vi "DPT Panel Dryer PreCondition.vi"(0 "Test Fixture Hardware":T1={"Power "={"Yokogawa"={"WT210"={"Sample Rate (1: 0.25s)"=1, "A Range (12: 20A)"=11, "V Range (6: 600V)"=4, "Power VISA Yokogawa WT210"="WT210"}, "WT500"={"Power VISA Yokogawa WT500"="", "V Range (8: 1000V)"=6, "I Range (7: 40A)"=7, "Update Rate (3: 500ms)"=2}, "WT310_2"={"Sample Rate (1: 0.25s)"=1, "A Range (12: 20A)"=11, "V Range (6: 600V)"=4, "Power VISA Yokogawa WT310_2"="WT310_2"}, "WT310_3"={"Sample Rate (1: 0.25s)"=1, "A Range (12: 20A)"=11, "V Range (6: 600V)"=4, "Power VISA Yokogawa WT310_3"="WT310_3"}}, "Aplus"={"Aplus IP Address"="192.168.1.101", "Remote Port"=502, "Instrument"="APLUS", "Instr Driver Revision"="1.03.0053"}, "Power Limits"={"Crest Factor"={"Upper Limit"=1.49, "Lower Limit"=1.34}, "Harmonic Content"={"Uthd"=2.0}, "Voltage"={"% Error"=2.0}, "Stability"={"<1 Watt "={"Wattage"=1.0, "Slope (mW/H)"=10.0}, ">1 Watt"={"1%Power/Hour"=1.0}}}, "Nominal Voltage"=120, "Time Limit (s)"=10800.0, "Power Variation Limit (%)"=50.0, "Power Supply"={"Chroma 61605"="CHROMA", "Use Chroma?"=FALSE}}, "Weight Scale"={"Com Options"={"IND560Scale VISA"="IND560", "IP Address"="", "Remote Port"=502, "Setra Scale VISA"="SETRA", "GSE 350"="GSE350"}, "Select Scale"=""}, "Flow Rates"={"Laurel Cold IP Address"="", "Laurel Hot IP Address"="", "Hot Water Laurel VISA"="LaurelMeter_Hot", "Cold Water Laurel VISA"="LaurelMeter_Cold", "Remote Port"=0, "Laurel Communication Type"="", "Meters To Collect (Hot Cold)"="", "HOT Laurel Reference"=refnum, "COLD Laurel Reference"=refnum}, "Analog Data"={"Agilent"={"Agilent 34972_1"="34972A_1", "Agilent 34972_2"="34972A_2", "Agilent 34972_3"="34972A_3", "Agilent 34972_4"="34972A_3", "Agilent 34972_5"="34972A_3", "Agilent 34972_6"="34972A_3", "Agilent Gain"=0.0, "TC Type (K,J,T)"="", "Instrument IDN?"="", "TC Channels-List"="", "Analog Channels-List"="", "Agilent Cluster Array"=[], "TC Channels-List 2"="", "Analog Channels-List 2"=""}, "Yokogawa"={"MW100"="MW100", "Intellifaucet"=FALSE}, "Select Analog"="", "TC Coefficients"={"TC Coefficients 1"=[], "TC Coefficients 2"=[], "TC Coefficients 3"=[], "TC Coefficients 4"=[], "TC Coefficients 5"=[], "TC Coefficients 6"=[], "TC Coefficients 7"=[]}, "NI Tasks (Dryer DOE)"=["TC Temps-Module 1", "TC Temps-Module 2", "TC Temps-Module 3", "TC Temps-Module 4", "TC Temps-Module 5", "Gas and Temp-Module 6", "AC_DC Events-Module 7"], "Laurel Analog"={"Laurel IP (Water Temp)"="", "Laurel IP (Pressure)"=""}}, "ITHX-Temp Humidity"={"IP Address 1"="", "Remote Port"=0, "IP Address 2"="", "IP Address 3"=""}, "Gas Meter COM Ports"={"Gas Meter 1"="COM3", "Gas Meter 2"="COM4", "Gas Meter 3"="COM5", "Gas Meter 4"="COM6", "Gas Meter 5"="COM7", "Gas Meter 6"="COM8"}, "Barometric Pressure"={"HEISE 901A"="HEISE", "Use Barometer?"=FALSE}} {"Power"."Yokogawa"."WT310_3"."V Range (6: 600V)" items=["Auto", "15V", "30V", "60V", "150V", "300V", "600V"]; "Power"."Yokogawa"."WT310_3"."A Range (12: 20A)" items=["Auto", "5mA", "10mA", "20mA", "50mA", "100mA", "200mA", "0.5A", "1A", "2A", "5A", "10A", "20A", "50mV", "100mV", "200mV", "2.5V", "5V", "10V"]; "Power"."Yokogawa"."WT310_3"."Sample Rate (1: 0.25s)" items=["0.1s", "0.25s", "0.5s", "1s", "2s", "5s"]; "Power"."Yokogawa"."WT310_2"."V Range (6: 600V)" items=["Auto", "15V", "30V", "60V", "150V", "300V", "600V"]; "Power"."Yokogawa"."WT310_2"."A Range (12: 20A)" items=["Auto", "5mA", "10mA", "20mA", "50mA", "100mA", "200mA", "0.5A", "1A", "2A", "5A", "10A", "20A", "50mV", "100mV", "200mV", "2.5V", "5V", "10V"]; "Power"."Yokogawa"."WT310_2"."Sample Rate (1: 0.25s)" items=["0.1s", "0.25s", "0.5s", "1s", "2s", "5s"]; "Power"."Yokogawa"."WT500"."Update Rate (3: 500ms)" items=["-", "100ms", "200ms", "500ms", "1s", "2s", "5s"]; "Power"."Yokogawa"."WT500"."I Range (7: 40A)" items=["AUTO", "500 mA", "1 A", "2 A", "5 A", "10 A", "20 A", "40 A", "S-AUTO", "50 mV", "100 mV", "200 mV", "500 mV", "1 V", "2 V", "5 V", "10 V", "250 mA", "500 mA", "1 A", "2.5 A", "5 A", "10 A", "20 A", "25 mV", "50 mV", "100 mV", "250 mV", "500 mV", "1 V", "2.5 V", "5 V"]; "Power"."Yokogawa"."WT500"."V Range (8: 1000V)" items=["AUTO", "15", "30", "60", "100", "150", "300", "600", "1000", "7.5", "15", "30", "50", "75", "150", "300", "500"]; "Power"."Yokogawa"."WT210"."V Range (6: 600V)" items=["Auto", "15V", "30V", "60V", "150V", "300V", "600V"]; "Power"."Yokogawa"."WT210"."A Range (12: 20A)" items=["Auto", "5mA", "10mA", "20mA", "50mA", "100mA", "200mA", "0.5A", "1A", "2A", "5A", "10A", "20A", "50mV", "100mV", "200mV", "2.5V", "5V", "10V"]; "Power"."Yokogawa"."WT210"."Sample Rate (1: 0.25s)" items=["0.1s", "0.25s", "0.5s", "1s", "2s", "5s"]}, 7 "Power On Threshold":dbl=25.0, 11 "Error In":errorcluster) -> (4 "Cold Dryer Weight":dbl, 15 "Error Out":errorcluster)   [LabVIEW 2018]
uses:
  Utility/Custom Pallet Controls/Custom Pallet String.ctl
  Utility/Custom Pallet Controls/Custom Pallet DBL.ctl
  Utility/Custom Pallet Controls/Custom Pallet Timer.ctl
  Washer DOE/Type Definitions/DOE Test Fixture Hardware.ctl
  Utility/Type Definitions/UTILITY Power Inputs Control.ctl
  Drivers/IND560 Scale Monitor/Type Definitions/IND560 Configuration.ctl
  Hybrid Water Heater/Type Definitions/HEWH Agilent Cluster.ctl
  Utility/Type Definitions/UTILITY TC Coefficients.ctl
  Drivers/Omega FMA-1600A Series Gas Flow Meter/Type Definitions/FMA1600A COM Ports.ctl
  Washer DOE/Type Definitions/DOE Dryer NI Card Settings.ctl
panel:
  out "RDB F":dbl(graph)
  in  "Tab Control":enum32{"Page 1", "Page 2"}(tab)
  out "15 min Up":bool
  out "Temp stable":bool
  out "Current State":string
  in  "Debug?":bool=TRUE
  in  "10 Min":i32=600
  in  "5min":dbl=300.0
  out "T0":dbl
  out "Tstart 5min":dbl
  out "Tstart 10min":dbl
  out "Debug State":string[](array[string])
  out "Power Greater Than Threshold":bool
  out "Timer":T7 format="%<%H:%M:%S>t"
  out "TC 1 - RDB (°F)":T8 format="%.2f"
  out "Ambient Temp(F)":T8 format="%.2f"
  out "Relative Humidity":T8 format="%.2f"
  out "Power (Watts)":T8 format="%.2f"
  out "Board ID":T9
  in  "Exit":bool
  # "Before any test cycle, operate the dryer without a test load in the non-heat mode for 15 minutes\nor until the discharge air temperature is varying less than 1 °F for 10 minutes, which ever is longer, in the test installation location\nwith the ambient conditions within the specified rest condition tolerances of 2.2."
  # "2.2 Ambient temperature and humidity. Maintain the room ambient air temperature at 75 ±3 °F and the room relative humidity at 50\n±10 percent relative humidity"
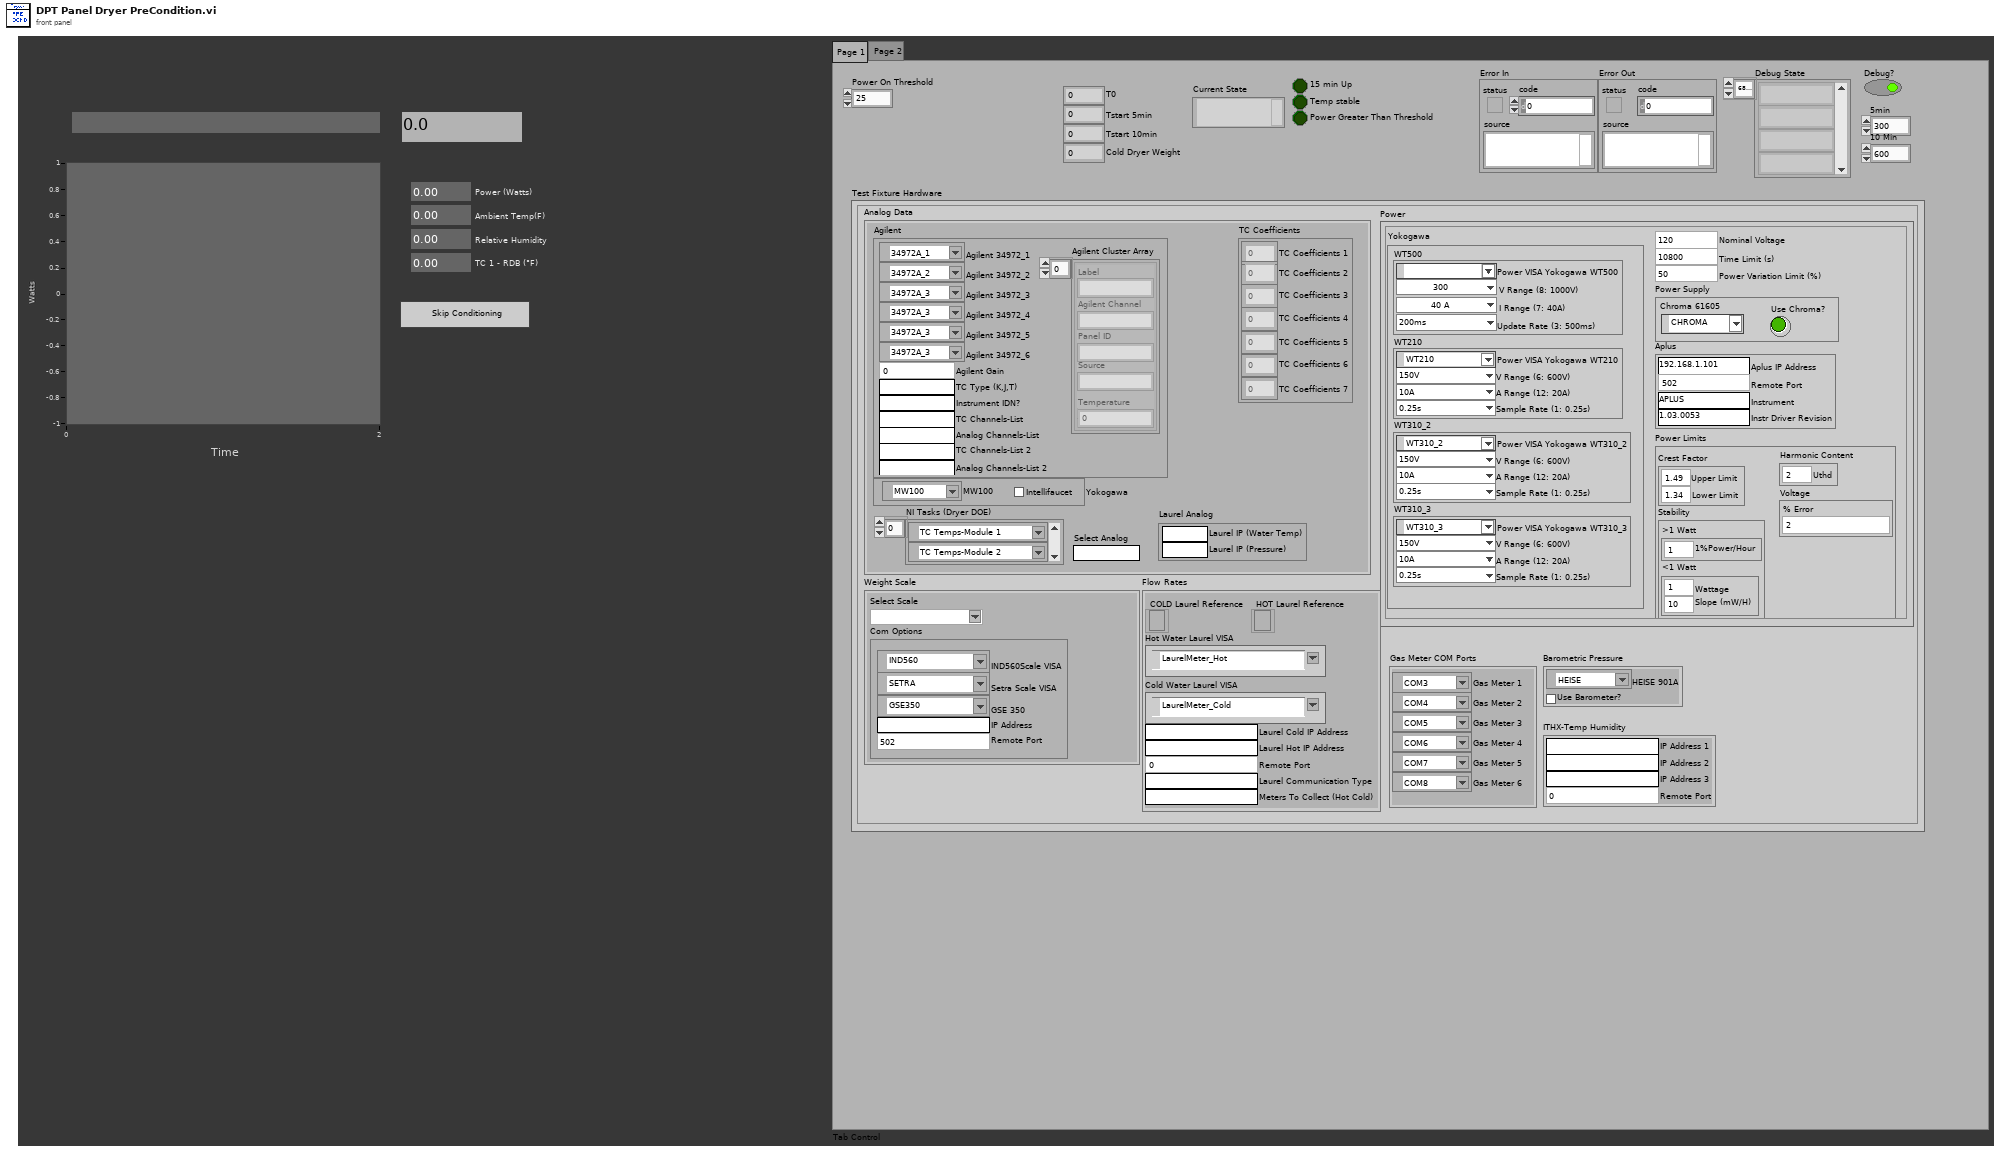
[diagram p1: front panel]
types:
  T1 = typedef "DOE Test Fixture Hardware.ctl" = cluster{"Power ":T2, "Weight Scale":cluster{"Com Options":T3, "Select Scale":string}, "Flow Rates":cluster{"Laurel Cold IP Address":string, "Laurel Hot IP Address":string, "Hot Water Laurel VISA":refnum<visa-resource-name>, "Cold Water Laurel VISA":refnum<visa-resource-name>, "Remote Port":u16, "Laurel Communication Type":string, "Meters To Collect (Hot Cold)":string, "HOT Laurel Reference":refnum<k5>, "COLD Laurel Reference":refnum<k5>}, "Analog Data":cluster{"Agilent":cluster{"Agilent 34972_1":refnum<visa-resource-name>, "Agilent 34972_2":refnum<visa-resource-name>, "Agilent 34972_3":refnum<visa-resource-name>, "Agilent 34972_4":refnum<visa-resource-name>, "Agilent 34972_5":refnum<visa-resource-name>, "Agilent 34972_6":refnum<visa-resource-name>, "Agilent Gain":dbl, "TC Type (K,J,T)":string, "Instrument IDN?":string, "TC Channels-List":string, "Analog Channels-List":string, "Agilent Cluster Array":T4[], "TC Channels-List 2":string, "Analog Channels-List 2":string}, "Yokogawa":cluster{"MW100":refnum<visa-resource-name>, "Intellifaucet":bool}, "Select Analog":string, "TC Coefficients":T5, "NI Tasks (Dryer DOE)":refnum<k21>[], "Laurel Analog":cluster{"Laurel IP (Water Temp)":string, "Laurel IP (Pressure)":string}}, "ITHX-Temp Humidity":cluster{"IP Address 1":string, "Remote Port":u16, "IP Address 2":string, "IP Address 3":string}, "Gas Meter COM Ports":T6, "Barometric Pressure":cluster{"HEISE 901A":refnum<visa-resource-name>, "Use Barometer?":bool}}
  T2 = typedef "UTILITY Power Inputs Control.ctl" = cluster{"Yokogawa":cluster{"WT210":cluster{"Sample Rate (1: 0.25s)":i32, "A Range (12: 20A)":i32, "V Range (6: 600V)":i32, "Power VISA Yokogawa WT210":refnum<visa-resource-name>}, "WT500":cluster{"Power VISA Yokogawa WT500":refnum<visa-resource-name>, "V Range (8: 1000V)":i32, "I Range (7: 40A)":i32, "Update Rate (3: 500ms)":i32}, "WT310_2":cluster{"Sample Rate (1: 0.25s)":i32, "A Range (12: 20A)":i32, "V Range (6: 600V)":i32, "Power VISA Yokogawa WT310_2":refnum<visa-resource-name>}, "WT310_3":cluster{"Sample Rate (1: 0.25s)":i32, "A Range (12: 20A)":i32, "V Range (6: 600V)":i32, "Power VISA Yokogawa WT310_3":refnum<visa-resource-name>}}, "Aplus":cluster{"Aplus IP Address":string, "Remote Port":i32, "Instrument":string, "Instr Driver Revision":string}, "Power Limits":cluster{"Crest Factor":cluster{"Upper Limit":dbl, "Lower Limit":dbl}, "Harmonic Content":cluster{"Uthd":dbl}, "Voltage":cluster{"% Error":dbl}, "Stability":cluster{"<1 Watt ":cluster{"Wattage":dbl, "Slope (mW/H)":dbl}, ">1 Watt":cluster{"1%Power/Hour":dbl}}}, "Nominal Voltage":i32, "Time Limit (s)":dbl, "Power Variation Limit (%)":dbl, "Power Supply":cluster{"Chroma 61605":refnum<visa-resource-name>, "Use Chroma?":bool}}
  T3 = typedef "IND560 Configuration.ctl" = cluster{"IND560Scale VISA":refnum<visa-resource-name>, "IP Address":string, "Remote Port":u16, "Setra Scale VISA":refnum<visa-resource-name>, "GSE 350":refnum<visa-resource-name>}
  T4 = typedef "HEWH Agilent Cluster.ctl" = cluster{"Label":string, "Agilent Channel":string, "Panel ID":string, "Source":string, "Temperature":dbl}
  T5 = typedef "UTILITY TC Coefficients.ctl" = cluster{"TC Coefficients 1":dbl[], "TC Coefficients 2":dbl[], "TC Coefficients 3":dbl[], "TC Coefficients 4":dbl[], "TC Coefficients 5":dbl[], "TC Coefficients 6":dbl[], "TC Coefficients 7":dbl[]}
  T6 = typedef "FMA1600A COM Ports.ctl" = cluster{"Gas Meter 1":refnum<visa-resource-name>, "Gas Meter 2":refnum<visa-resource-name>, "Gas Meter 3":refnum<visa-resource-name>, "Gas Meter 4":refnum<visa-resource-name>, "Gas Meter 5":refnum<visa-resource-name>, "Gas Meter 6":refnum<visa-resource-name>}
  T7 = typedef "Custom Pallet Timer.ctl" = dbl
  T8 = typedef "Custom Pallet DBL.ctl" = dbl
  T9 = typedef "Custom Pallet String.ctl" = string
  T10 = enum32{"invalid app kind", "Development System", "Run Time System", "Student Edition", "Embedded LabVIEW", "Evaluation", "Custom"}
  T11 = enum32{"Invalid", "Standard", "Closed", "Hidden", "Minimized", "Maximized"}
  T12 = typedef "DOE Dryer NI Card Settings.ctl" = cluster{"Disable NI Card 1":bool, "Disable NI Card 2":bool, "Disable NI Card 3":bool, "Disable NI Card 4":bool, "Disable NI Card 5":bool, "Disable NI Card 6":bool, "Disable NI Card 7":bool}
  T13 = cluster{"Core":cluster{"Current VI Reference":refnum<vi>, "Close Panel on Exit?":bool}, "Agilent Channel List":string, "Power On Threshold":dbl, "T0":dbl, "Tstart":dbl, "Temps":dbl[], "Test Fixture Hardware":T1}
  T14 = cluster{"Current VI Reference":refnum<vi>, "Close Panel on Exit?":bool}
  T15 = typedef "UTILITY Power Data.ctl" = cluster{"Current (A):Element 1":dbl, "Current (A):Element 2":dbl, "Power (W):Sigma":dbl, "Watt Hours (Wh):Sigma":dbl, "Voltage (V):Element 2":dbl, "Voltage (V):Element 1":dbl, "Current Crest Factor:Element 1":dbl, "Current Crest Factor:Element 2":dbl, "Voltage Harmonic (%):Element 1":dbl, "Voltage Harmonic (%):Element 2":dbl, "Voltage Crest Factor:Element 1":dbl, "Voltage Crest Factor:Element 2":dbl, "Time:Element 1":dbl, "Frequency (Hz):Element 1":dbl, "Apparent Power (VA):Element 1":dbl, "Apparent Power (VA):Element 2":dbl, "Power Factor:Element 1":dbl, "Power Factor:Element 2":dbl, "Max Watt Hours":dbl, "Voltage (V):Element 2 Avg":dbl, "Voltage (V):Element 1 Avg":dbl}
  T16 = typedef "iBTHX Data Values.ctl" = cluster{"iBTHX Barometric Pressure (mbar/hPa)":dbl, "iBTHX Humidity (%)":dbl, "iBTHX Temperature (°F)":dbl, "iBTHX DewPoint Temp":dbl}
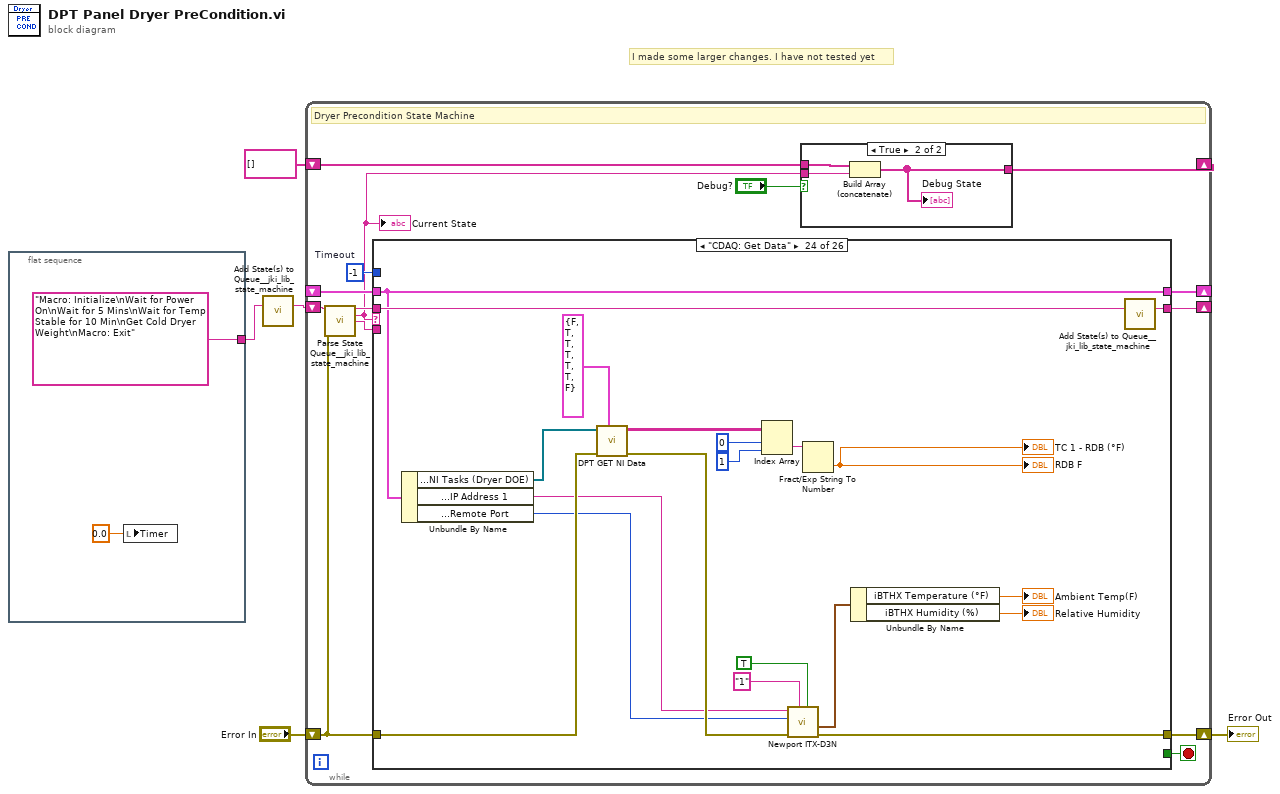
[diagram p0: block diagram]
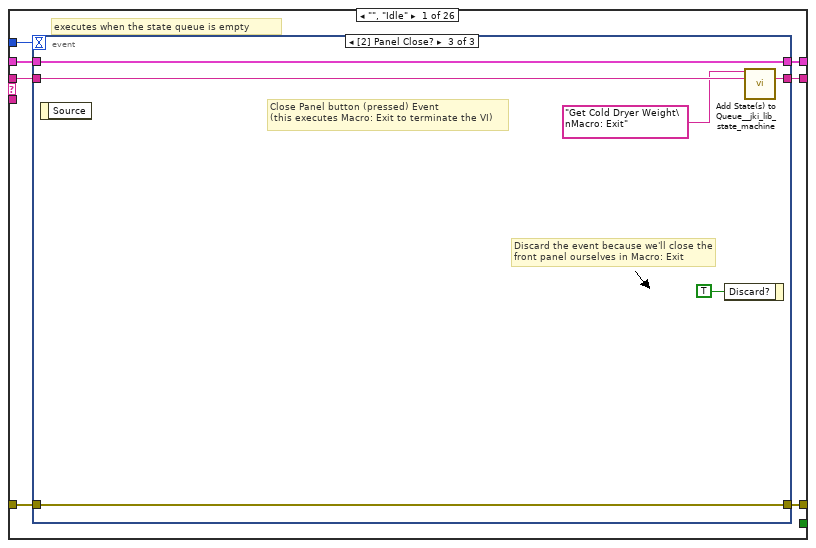
[diagram p3: hidden frame]
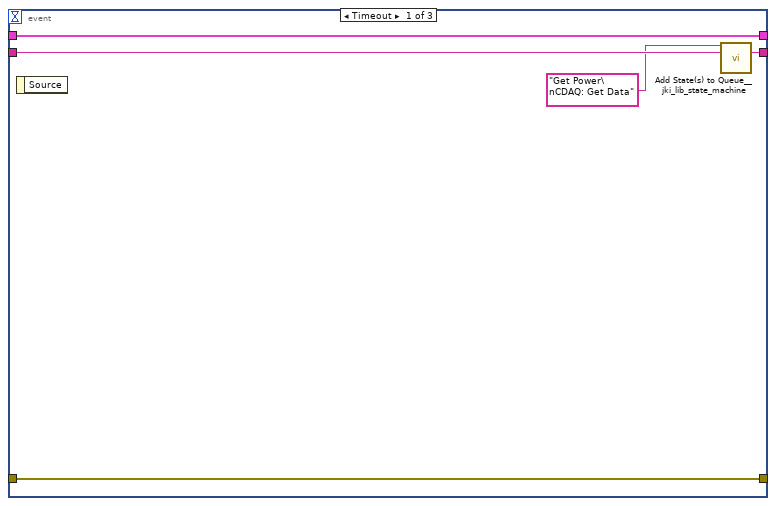
[diagram p4: hidden frame]
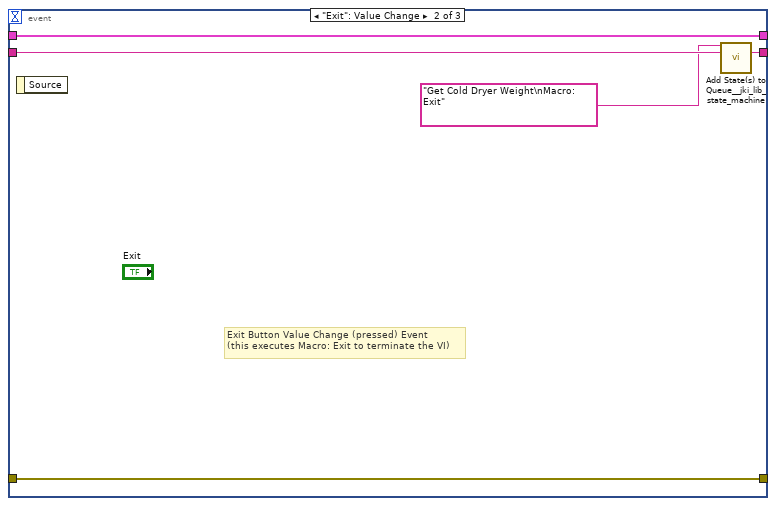
[diagram p5: hidden frame]
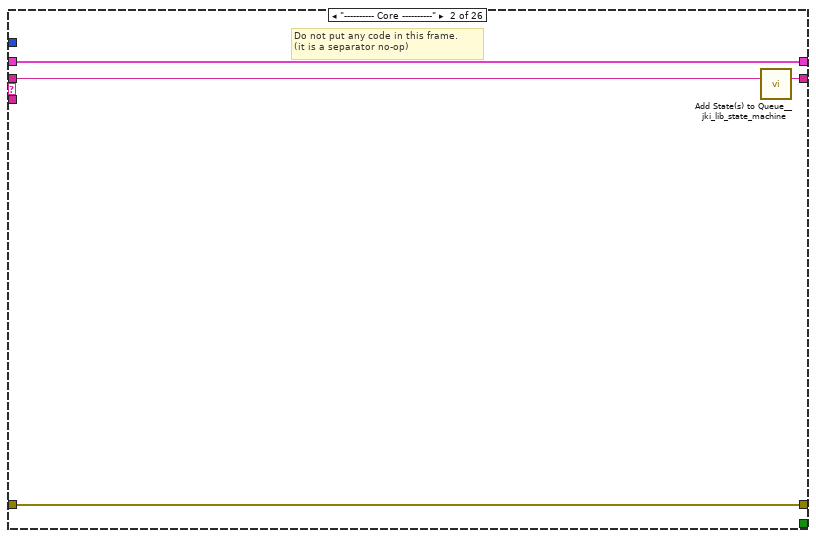
[diagram p6: hidden frame]
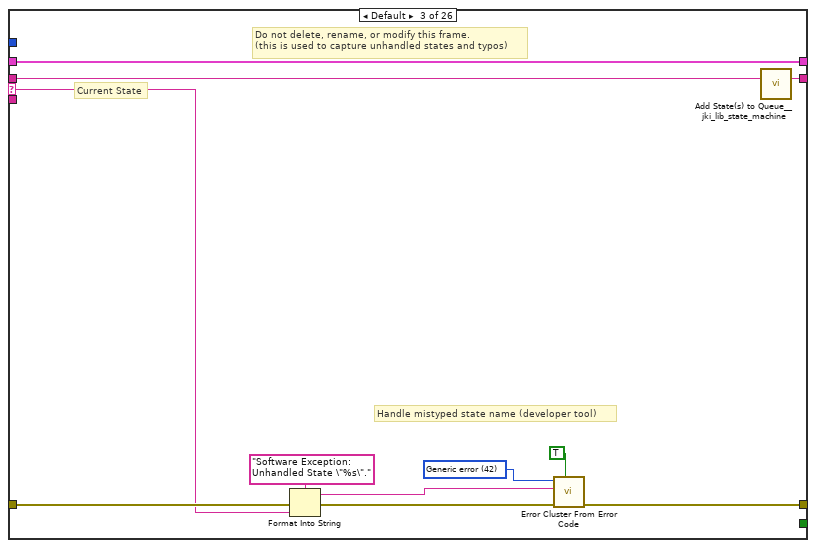
[diagram p7: hidden frame]
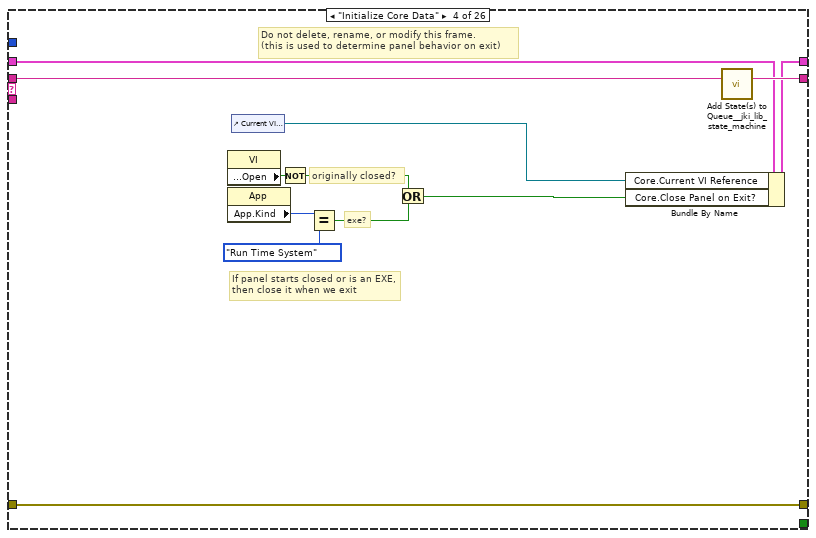
[diagram p8: hidden frame]
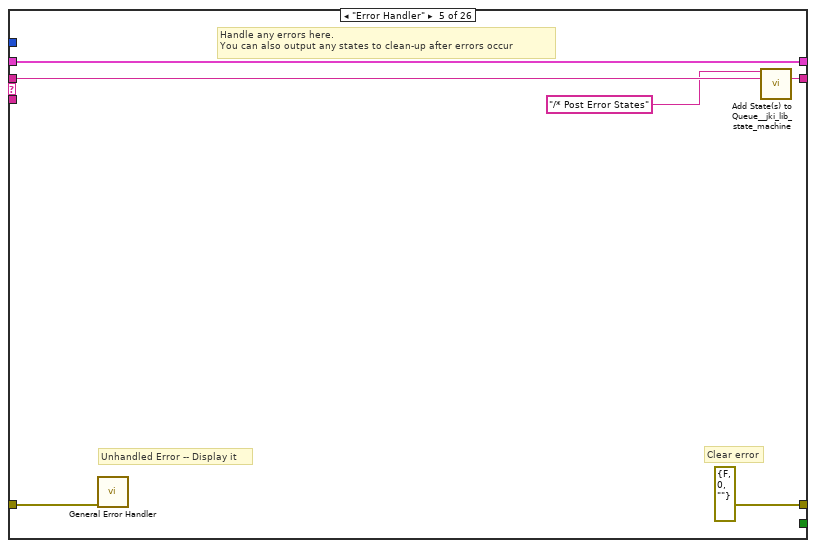
[diagram p9: hidden frame]
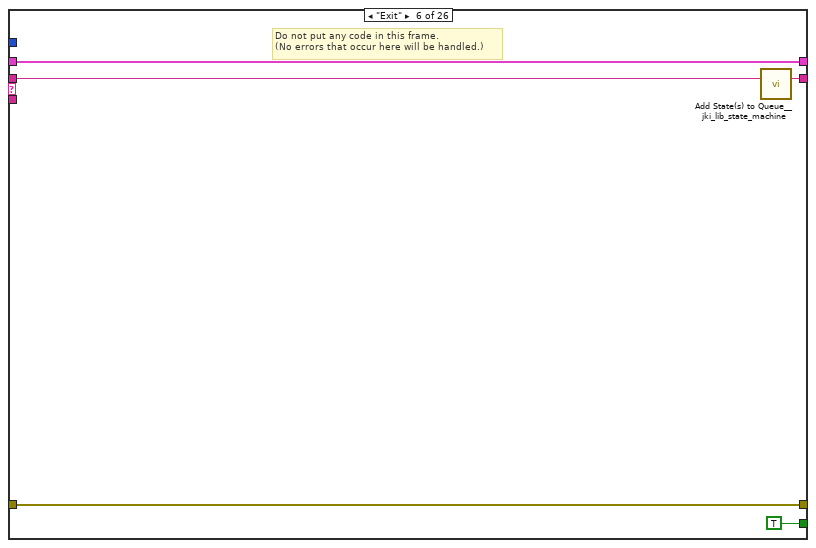
[diagram p10: hidden frame]
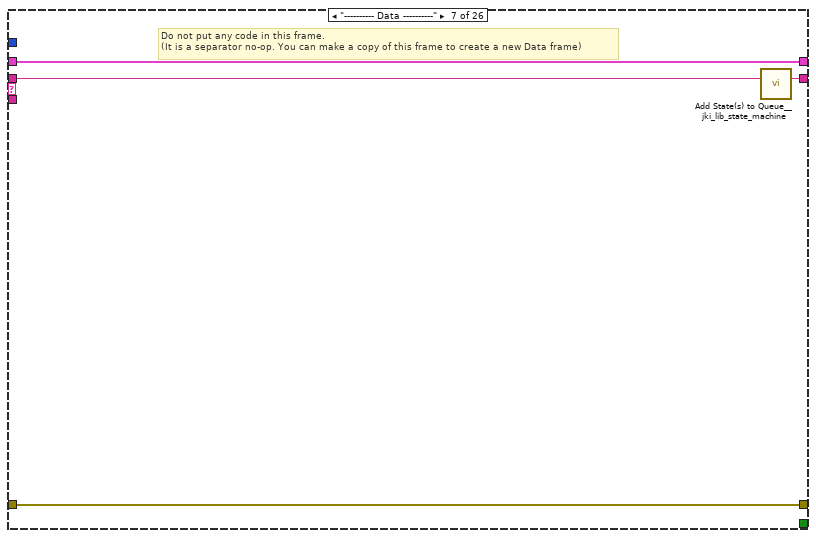
[diagram p11: hidden frame]
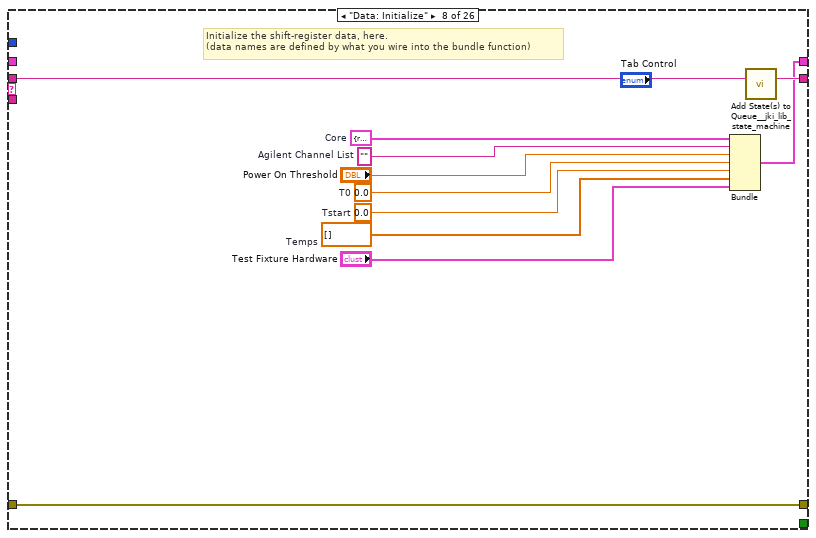
[diagram p12: hidden frame]
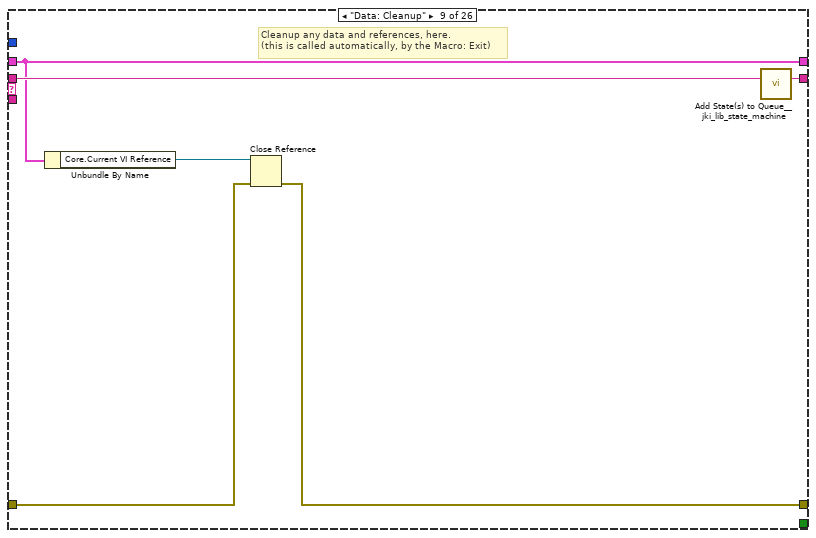
[diagram p13: hidden frame]
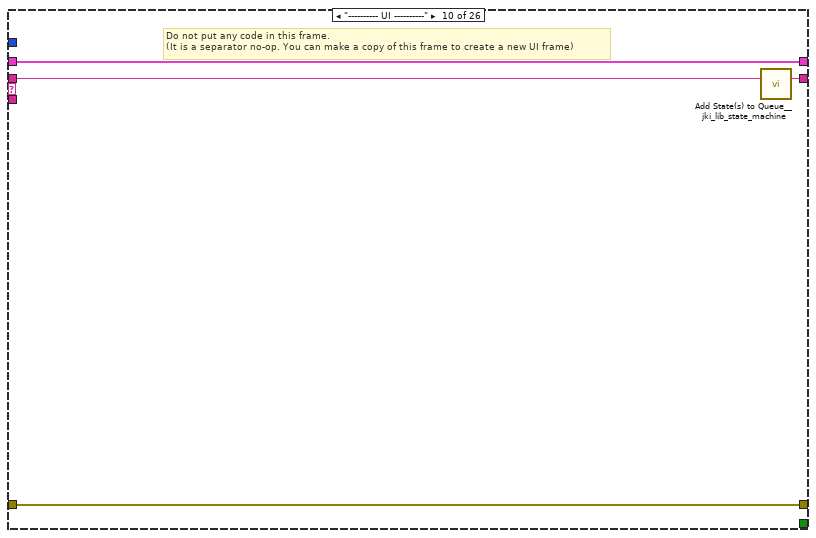
[diagram p14: hidden frame]
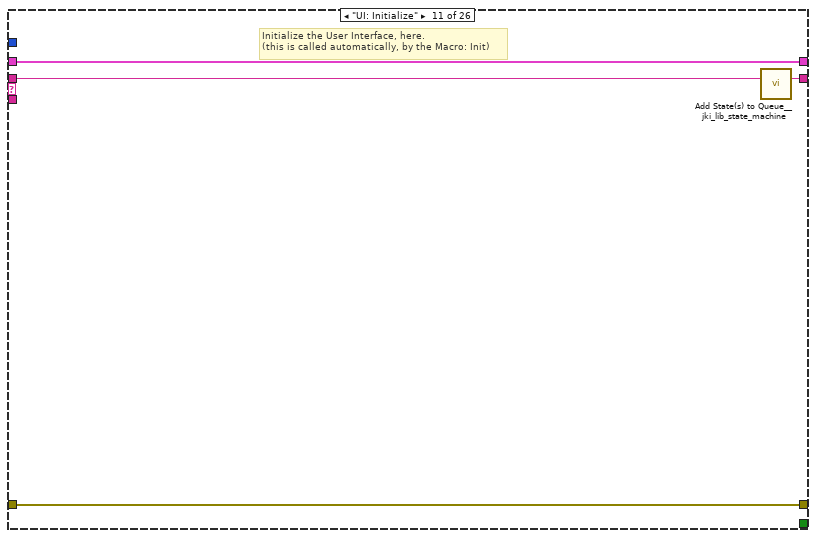
[diagram p15: hidden frame]
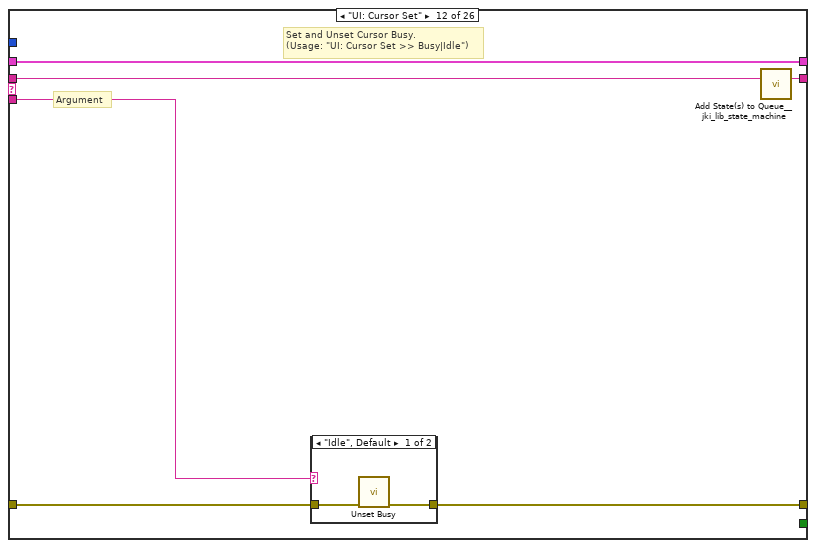
[diagram p16: hidden frame]
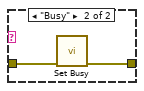
[diagram p17: hidden frame]
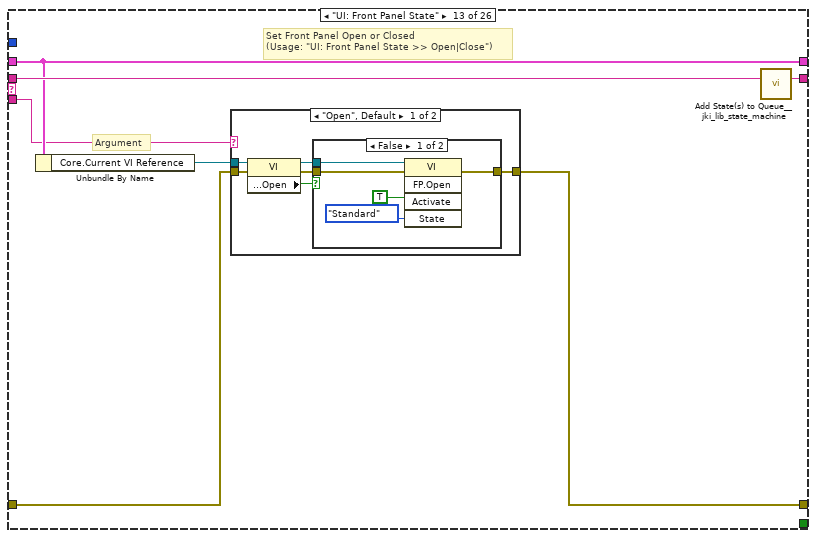
[diagram p18: hidden frame]
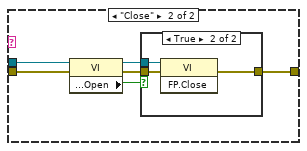
[diagram p20: hidden frame]
diagram:
  # "I made some larger changes. I have not tested yet"
  n1 = flat-sequence {
    tunnel: ["Macro: Initialize\nWait for Power On\nWait for 5 Mins\nWait for Temp Stable for 10 Min\nGet Cold Dryer Weight\nMacro: Exit"] -> w4
    frame #0 {
      n2 = local write "Timer"(0.0 ("Timer")) -> ()
    }
  }
  n3 = call <vilib>:"Add State(s) to Queue__jki_lib_state_machine.vi"("State(s) in (\"\")"=w4) -> ("States Out"=w5:string)  [unwired: 14 in]
  n4 = while {
    shift-right: [w16] -> _
    shift-left: _ -> [w15]
    shift-right: [w18] -> w2
    shift-left: "Error In" -> [w13]
    shift-right: [w8] -> _
    shift-left: w5 -> [w19]
    shift-right: [w10] -> _
    shift-left: string[] [] -> [w9]
    stop <- w17 stop-if-true
    w14 = -1  # Timeout
    # "Dryer Precondition State Machine"
    n5 = call <vilib>:"Parse State Queue__jki_lib_state_machine.vi"("State Queue"=w19, "Error In (no error)"=w13) -> ("Remaining States"=w21:string, "Current State"=w11:string, "Arguments"=w20:string)  [unwired: 11 in]
    "Current State" <- w11
    n6 = case shown="\"CDAQ: Get Data\"" w11 {
      selector: w11 -> [_ _ w53 _ _ _ _ _ _ _ _ _ _ _ _ _ _ _ _ _ _ _ _ _ _ _]
      tunnel: w21 -> [w32 w52 w57 w75 w81 w86 w90 w101 w107 w111 w115 w121 w132 w158 w163 w173 w177 w188 w211 w235 w264 w271 w279 w299 w306 w315]
      tunnel: w20 -> [_ _ _ _ _ _ _ _ _ _ _ w116 w126 _ _ _ _ _ _ _ _ _ _ _ _ _]
      tunnel: w15 -> [w30 w49 w55 w66 w78 w84 w87 _ w103 w108 w113 w119 w128 w155 w160 w170 w174 w184 w208 w232 w261 w266 w277 w297 w304 w307]
      tunnel: [w29 w50 w59 w72 errorcluster {"status"=FALSE, "code"=0, "source"=""} ("error out") w83 w88 w99 w104 w109 w112 w117 w129 w156 w161 w171 w175 w185 w209 w233 w262 w267 w272 w288 w300 w308] -> w18
      tunnel: w13 -> [w28 w50 w58 w72 w77 w83 w88 w99 w102 w109 w112 w118 w130 w156 w161 w171 w175 w185 w209 w233 w262 w265 w273 w295 w300 w309]
      tunnel: [w31 w51 w56 w74 w80 w85 w89 w100 w106 w110 w114 w120 w131 w157 w162 w172 w176 w187 w210 w234 w263 w270 w278 w298 w305 w314] -> w8
      tunnel: [_ _ _ _ _ TRUE _ _ _ _ _ _ _ _ _ _ _ _ _ _ _ _ _ _ _ _] -> w17
      tunnel: [w27 w49 w55 w73 w78 w84 w87 w95 w103 w108 w113 w119 w128 w155 w160 w170 w174 w183 w207 w231 w261 w269 w277 w297 w304 w307] -> w16
      tunnel: w14 -> [w26 _ _ _ _ _ _ _ _ _ _ _ _ _ _ _ _ _ _ _ _ _ _ _ _ _]
      frame "", "Idle" {
        # "executes when the state queue is empty"
        n7 = event shown="[2] Panel Close?" {
          selector: _ -> [_ _ _]
          dyn-events: _ -> [_ _ _]
          timeout: w26 -> [_ _ _]
          tunnel: w32 -> [w37 w42 w48]
          tunnel: [w36 w41 w47] -> w31
          tunnel: w30 -> [w33 w38 w45]
          tunnel: [w35 w40 w46] -> w29
          tunnel: w28 -> [w35 w40 w46]
          tunnel: [w33 w38 w45] -> w27
          event Timeout {
            n8 = event-data() -> ()  [unwired: 1 in, 1 out]
            n9 = call <vilib>:"Add State(s) to Queue__jki_lib_state_machine.vi"("State(s) in Front (\"\")"="Get Power\nCDAQ: Get Data" ("State(s) in Front (\"\")"), "State(s) in (\"\")"=w37) -> ("States Out"=w36:string)  [unwired: 13 in]
          }
          event "Exit": Value Change {
            # "Exit Button Value Change (pressed) Event\n(this executes Macro: Exit to terminate the VI)"
            n10 = event-data() -> ()  [unwired: 1 in, 1 out]
            n11 = call <vilib>:"Add State(s) to Queue__jki_lib_state_machine.vi"("State(s) in Front (\"\")"="Get Cold Dryer Weight\nMacro: Exit", "State(s) in (\"\")"=w42) -> ("States Out"=w41:string)  [unwired: 13 in]
          }
          event Panel Close? {
            # "Discard the event because we'll close the front panel ourselves in Macro: Exit"
            # "Close Panel button (pressed) Event\n(this executes Macro: Exit to terminate the VI)"
            n12 = event-data() -> ()  [unwired: 1 in, 1 out]
            n13 = event-data("Discard?"=TRUE) -> ()  [unwired: 1 in, 1 out]
            n14 = call <vilib>:"Add State(s) to Queue__jki_lib_state_machine.vi"("State(s) in Front (\"\")"="Get Cold Dryer Weight\nMacro: Exit", "State(s) in (\"\")"=w48) -> ("States Out"=w47:string)  [unwired: 13 in]
          }
        }
      }
      frame "---------- Core ----------" {
        # "Do not put any code in this frame.\n(it is a separator no-op)"
        n15 = call <vilib>:"Add State(s) to Queue__jki_lib_state_machine.vi"("State(s) in (\"\")"=w52) -> ("States Out"=w51:string)  [unwired: 14 in]
      }
      frame Default {
        w62 = 42 items=["No error", "Argument error", "Memory is full", "Out of zone", "End of file", "File already open", "Generic file I/O error", "File not found", "File permission error", "Disk is full", "Duplicate path", "Too many files open", "System feature not enabled", "Resource file not found", "Cannot add resource", "Resource not found", "Image not found", "Image memory error", "Pen does not exist", "Config type invalid", "Config token not found", "Config parse error", "Config memory error", "Bad external code format", "Bad external code offset", "External code not present", "Null window", "Destroy window error", "Null menu", "Print aborted", "Bad print record", "Print driver error", "Windows error during printing", "Memory error during printing", "Print dialog error", "Generic print error", "Invalid device refnum", "Device not found", "Device parameter error", "Device unit error", "Cannot open device", "Device call aborted", "Generic error", "Cancelled by user", "Object ID too low", "Object ID too high", "Object not in heap", "Unknown heap", "Unknown object (invalid DefProc)", "Unknown object (DefProc not in table)", "Message out of range", "Invalid (null) method", "Unknown message", "Manager call not supported", "Bad address", "Network operation in progress", "Network operation timed out", "Connection is busy", "Network attribute not supported", "Network error", "Address in use", "System out of memory", "Connection aborted", "Connection refused", "Not connected", "Already connected", "Connection closed", "Initialization error (interapplication manager)", "Bad occurrence", "Wait on unbound occurrence handler", "Occurrence queue overflow", "Datalog type conflict", "Unused", "Unrecognized type (interapplication manager)", "Memory corrupt", "Failed to make temporary DLL", "Old CIN version", "Drag socket not found", "Failed to load drop-object", "Failed to register OLE object", "Failed to release OLE object", "Format specifier type mismatch", "Unknown format specifier", "Too few format specifiers", "Too many format specifiers", "Scan failed", "Newer CIN version", "Error converting to variant", "Runtime menu error", "Password tampered", "Variant attribute not found", "Incompatible variant data type", "Event data is not available", "Event Store is not present", "Occurrence is not found", "Event Queue is not created", "Event info is not available", "Refnum passed is NULL", "Error retrieving Class GUID", "Error retrieving CoClass GUID", "Error retrieving TypeLib GUID.", "Bad built application magic bytes.", "Specific driver is different from the specific driver associated with the Logical Name.", "There is no session opened to the class driver.", "Max Error", "MAX - Error with config objects", "MAX - Error loading configuration", "MAX - Group not supported"]
        # "Current State"
        # "Do not delete, rename, or modify this frame.\n(this is used to capture unhandled states and typos)"
        # "Handle mistyped state name (developer tool)"
        n16 = Format Into String(format string="Software Exception: Unhandled State \"%s\"." ("message"), error in=w58, w53) -> (resulting string=w61:string, error out=w60:errorcluster)  [unwired: 1 in]
        n17 = call <vilib>:"Error Cluster From Error Code.vi"("show call chain? (False)"=TRUE, "error in (no error)"=w60, "error message (\"\")"=w61, "error code (0)"=w62) -> ("error out"=w59:errorcluster)  [unwired: 5 in]
        n18 = call <vilib>:"Add State(s) to Queue__jki_lib_state_machine.vi"("State(s) in (\"\")"=w57) -> ("States Out"=w56:string)  [unwired: 14 in]
      }
      frame "Initialize Core Data" {
        # "Do not delete, rename, or modify this frame.\n(this is used to determine panel behavior on exit)"
        # "originally closed?"
        # "exe?"
        # "If panel starts closed or is an EXE, then close it when we exit"
        n19 = property class="VI"() -> ("Front Panel.Open"=w71:bool)  [unwired: 2 in, 2 out]
        n20 = property class="App"() -> ("App.Kind"=w70:T10)  [unwired: 2 in, 2 out]
        n21 = control-ref of="Current VI Reference"() -> (w64:refnum<vi>)
        n22 = Not(x=w71) -> (.not. x?=w68:bool)
        n23 = Equal?(x=w70, y=T10."Run Time System" ("Application:Kind")) -> (x = y?=w67:bool)
        n24 = Or(x=w68, y=w67) -> (x .or. y?=w65:bool)
        n25 = Bundle By Name(cluster=w66, "Core.Current VI Reference"=w64, "Core.Close Panel on Exit?"=w65) -> (w73:T13)
        n26 = call <vilib>:"Add State(s) to Queue__jki_lib_state_machine.vi"("State(s) in (\"\")"=w75) -> ("States Out"=w74:string)  [unwired: 14 in]
      }
      frame "Error Handler" {
        # "Unhandled Error -- Display it"
        # "Handle any errors here.\nYou can also output any states to clean-up after errors occur"
        # "Clear error"
        n27 = call <vilib>:"General Error Handler.vi"("error in (no error)"=w77) -> ()  [unwired: 10 in, 5 out]
        n28 = call <vilib>:"Add State(s) to Queue__jki_lib_state_machine.vi"("State(s) in Front (\"\")"="/* Post Error States", "State(s) in (\"\")"=w81) -> ("States Out"=w80:string)  [unwired: 13 in]
      }
      frame "Exit" {
        # "Do not put any code in this frame.\n(No errors that occur here will be handled.)"
        n29 = call <vilib>:"Add State(s) to Queue__jki_lib_state_machine.vi"("State(s) in (\"\")"=w86) -> ("States Out"=w85:string)  [unwired: 14 in]
      }
      frame "---------- Data ----------" {
        # "Do not put any code in this frame.\n(It is a separator no-op. You can make a copy of this frame to create a new Data frame)"
        n30 = call <vilib>:"Add State(s) to Queue__jki_lib_state_machine.vi"("State(s) in (\"\")"=w90) -> ("States Out"=w89:string)  [unwired: 14 in]
      }
      frame "Data: Initialize" {
        w92 = dbl[] []  # Temps
        w93 = 0.0  # Tstart
        w94 = 0.0  # T0
        w96 = ""  # Agilent Channel List
        w98 = T14 {"Current VI Reference"=refnum, "Close Panel on Exit?"=TRUE}  # Core
        # "Initialize the shift-register data, here.\n(data names are defined by what you wire into the bundle function)"
        n31 = Bundle("Core"=w98, "Agilent Channel List"=w96, "Power On Threshold"="Power On Threshold", "T0"=w94, "Tstart"=w93, "Temps"=w92, "Test Fixture Hardware"="Test Fixture Hardware") -> (w95:T13)  [unwired: 1 in]
        n32 = call <vilib>:"Add State(s) to Queue__jki_lib_state_machine.vi"("State(s) in (\"\")"=w101) -> ("States Out"=w100:string)  [unwired: 14 in]
      }
      frame "Data: Cleanup" {
        # "Cleanup any data and references, here.\n(this is called automatically, by the Macro: Exit)"
        n33 = Unbundle By Name(w103) -> ("Core.Current VI Reference"=w105:refnum<vi>)
        n34 = Close Reference(reference=w105, error in (no error)=w102) -> (error out=w104:errorcluster)
        n35 = call <vilib>:"Add State(s) to Queue__jki_lib_state_machine.vi"("State(s) in (\"\")"=w107) -> ("States Out"=w106:string)  [unwired: 14 in]
      }
      frame "---------- UI ----------" {
        # "Do not put any code in this frame.\n(It is a separator no-op. You can make a copy of this frame to create a new UI frame)"
        n36 = call <vilib>:"Add State(s) to Queue__jki_lib_state_machine.vi"("State(s) in (\"\")"=w111) -> ("States Out"=w110:string)  [unwired: 14 in]
      }
      frame "UI: Initialize" {
        # "Initialize the User Interface, here.\n(this is called automatically, by the Macro: Init)"
        n37 = call <vilib>:"Add State(s) to Queue__jki_lib_state_machine.vi"("State(s) in (\"\")"=w115) -> ("States Out"=w114:string)  [unwired: 14 in]
      }
      frame "UI: Cursor Set" {
        # "Argument"
        # "Set and Unset Cursor Busy.\n(Usage: \"UI: Cursor Set >> Busy|Idle\")"
        n38 = case shown="\"Idle\", Default" w116 {
          tunnel: w118 -> [w123 w125]
          tunnel: [w122 w124] -> w117
          frame "Idle", Default {
            n39 = call <vilib>:"Unset Busy.vi"("error in (no error)"=w123) -> ("error out"=w122:errorcluster)  [unwired: 10 in]
          }
          frame "Busy" {
            n40 = call <vilib>:"Set Busy.vi"("error in (no error)"=w125) -> ("error out"=w124:errorcluster)  [unwired: 9 in, 1 out]
          }
        }
        n41 = call <vilib>:"Add State(s) to Queue__jki_lib_state_machine.vi"("State(s) in (\"\")"=w121) -> ("States Out"=w120:string)  [unwired: 14 in]
      }
      frame "UI: Front Panel State" {
        # "Argument"
        # "Set Front Panel Open or Closed\n(Usage: \"UI: Front Panel State >> Open|Close\")"
        n42 = Unbundle By Name(w128) -> ("Core.Current VI Reference"=w127:refnum<vi>)
        n43 = case shown="\"Open\", Default" w126 {
          tunnel: w130 -> [w136 w149]
          tunnel: [w138 w150] -> w129
          tunnel: w127 -> [w137 w147]
          frame "Open", Default {
            n44 = property class="VI"(reference=w137, error in=w136) -> (reference out=w134:refnum<vi>, error out=w135:errorcluster, "Front Panel.Open"=w133:bool)
            n45 = case shown="False" w133 {
              tunnel: [w141 w144] -> w138
              tunnel: w135 -> [w140 w144]
              tunnel: w134 -> [w139 _]
              frame False {
                n46 = invoke class="VI" method="FP.Open"(reference=w139, error in=w140, "Activate"=TRUE, "State"=T11."Standard") -> (error out=w141:errorcluster)  [unwired: 1 in, 4 out]
              }
              frame True {
              }
            }
          }
          frame "Close" {
            n47 = property class="VI"(reference=w147, error in=w149) -> (reference out=w146:refnum<vi>, error out=w148:errorcluster, "Front Panel.Open"=w145:bool)
            n48 = case shown="True" w145 {
              tunnel: [w151 w154] -> w150
              tunnel: w148 -> [w151 w153]
              tunnel: w146 -> [_ w152]
              frame False {
              }
              frame True {
                n49 = invoke class="VI" method="FP.Close"(reference=w152, error in=w153) -> (error out=w154:errorcluster)  [unwired: 1 in, 2 out]
              }
            }
          }
        }
        n50 = call <vilib>:"Add State(s) to Queue__jki_lib_state_machine.vi"("State(s) in (\"\")"=w132) -> ("States Out"=w131:string)  [unwired: 14 in]
      }
      frame "---------- Macro ----------" {
        # "Do not put any code in this frame.\n(It is a separator no-op. You can make a copy of this frame to create a new Macro frame)"
        n51 = call <vilib>:"Add State(s) to Queue__jki_lib_state_machine.vi"("State(s) in (\"\")"=w158) -> ("States Out"=w157:string)  [unwired: 14 in]
      }
      frame "Macro: Initialize" {
        w159 = "Data: Initialize\nInit: Time\nInitialize Core Data\nUI: Initialize\nUI: Front Panel State >> Open"  # Data: Initialize Init: Time Initialize Core Data UI: Initialize UI: Front Panel State >> Open
        # "Initialization Macro\n(This is called once, when the VI starts)"
        n52 = call <vilib>:"Add State(s) to Queue__jki_lib_state_machine.vi"("State(s) in Front (\"\")"=w159, "State(s) in (\"\")"=w163) -> ("States Out"=w162:string)  [unwired: 13 in]
      }
      frame "Macro: Exit" {
        # "Exit Macro\n(This is called once, when the VI exits)"
        n53 = Unbundle By Name(w170) -> ("Core.Close Panel on Exit?"=w169:bool)
        n54 = Select(t="UI: Front Panel State >> Close", s=w169, f="") -> (s? t:f=w166:string)
        n55 = call <vilib>:"Add State(s) to Queue__jki_lib_state_machine.vi"("State(s) in (\"\")"=w166, "State(s) at Back (\"\")"="Data: Cleanup\nExit") -> ("States Out"=w164:string)  [unwired: 13 in]
        n56 = call <vilib>:"Add State(s) to Queue__jki_lib_state_machine.vi"("State(s) in Front (\"\")"=w164, "State(s) in (\"\")"=w173) -> ("States Out"=w172:string)  [unwired: 13 in]
      }
      frame "----------Test ----------" {
        # "Template Separator\n(You can make a copy of, or modify, this frame)"
        n57 = call <vilib>:"Add State(s) to Queue__jki_lib_state_machine.vi"("State(s) in (\"\")"=w177) -> ("States Out"=w176:string)  [unwired: 14 in]
      }
      frame "Wait for Power On" {
        n58 = local read "Power (Watts)"() -> (w179:T8)
        n59 = Unbundle By Name(w184) -> ("Tstart"=w181:dbl, "Power On Threshold"=w180:dbl)
        n60 = Greater?(x=w180, y=w179) -> (0:w178:bool)
        "Power Greater Than Threshold" <- w178
        n61 = case shown="True" w178 {
          tunnel: w184 -> [w190 w198]
          tunnel: [w190 w197] -> w183
          tunnel: ["" ("State(s) in Front (\"\")") w195] -> w182
          tunnel: w181 -> [_ _]
          frame False {
          }
          frame True {
            n62 = call "UTILITY E-Time.vi"() -> ("Elapsed Time (sec)"=w191:dbl)  [unwired: 9 in, 2 out]
            n63 = call "UTILITY Timeout Calc.vi"("Timer"=w191, "Gather Data Period"=1000) -> ("coerced(x)"=w194:i32)  [unwired: 8 in, 1 out]
            n64 = event shown="[0] Timeout" {
              selector: _ -> [_]
              dyn-events: _ -> [_]
              timeout: w194 -> [_]
              tunnel: [w199] -> w196
              tunnel: ["Get Power\nCDAQ: Get Data\nWait for Power On" ("State(s) in Front (\"\")")] -> w195
              tunnel: [w199] -> w192
              event Timeout {
                n65 = event-data() -> ()  [unwired: 1 in, 2 out]
                n66 = call "UTILITY E-Time.vi"() -> ("Elapsed Time (sec)"=w199:dbl)  [unwired: 9 in, 2 out]
              }
            }
            n67 = Bundle By Name(cluster=w198, "Tstart"=w196, "T0"=w192) -> (w197:T13)
          }
        }
        n68 = call <vilib>:"Add State(s) to Queue__jki_lib_state_machine.vi"("State(s) in Front (\"\")"=w182, "State(s) in (\"\")"=w188) -> ("States Out"=w187:string)  [unwired: 13 in]
        "Board ID" <- "Start Fluffing: Waiting for Power ON"
      }
      frame "Wait for 5 Mins" {
        n69 = Unbundle By Name(w208) -> ("Tstart"=w205:dbl)
        n70 = local read "Timer"() -> (w203:T7)
        n71 = Greater?(x=w203, y="5min") -> (0:w204:bool)
        n72 = case shown="False" w204 {
          tunnel: w208 -> [w218 w222]
          tunnel: [w217 w222] -> w207
          tunnel: [w215 "" ("State(s) in Front (\"\")")] -> w206
          tunnel: w205 -> [_ _]
          frame False {
            n73 = call "UTILITY E-Time.vi"() -> ("Elapsed Time (sec)"=w212:dbl)  [unwired: 9 in, 2 out]
            n74 = call "UTILITY Timeout Calc.vi"("Timer"=w212, "Gather Data Period"=1000) -> ("coerced(x)"=w214:i32)  [unwired: 8 in, 1 out]
            n75 = event shown="[0] Timeout" {
              selector: _ -> [_]
              dyn-events: _ -> [_]
              timeout: w214 -> [_]
              tunnel: [w220] -> w216
              tunnel: ["Post Time\nGet Power\nCDAQ: Get Data\nWait for 5 Mins" ("State(s) in Front (\"\")")] -> w215
              event Timeout {
                n76 = event-data() -> ()  [unwired: 1 in, 2 out]
                n77 = call "UTILITY E-Time.vi"() -> ("Elapsed Time (sec)"=w220:dbl)  [unwired: 9 in, 2 out]
              }
            }
            "Tstart 5min" <- w216
            n78 = Bundle By Name(cluster=w218, "Tstart"=w216) -> (w217:T13)
          }
          frame True {
          }
        }
        n79 = local write "Board ID"("Air Fluffing...") -> ()
        n80 = call <vilib>:"Add State(s) to Queue__jki_lib_state_machine.vi"("State(s) in Front (\"\")"=w206, "State(s) in (\"\")"=w211) -> ("States Out"=w210:string)  [unwired: 13 in]
      }
      frame "Wait for Temp Stable for 10 Min" {
        n81 = Unbundle By Name(w232) -> ("Tstart"=w229:dbl, "Temps"=w223:dbl[])
        n82 = Array Size(array=w223) -> (size(s)=w227:i32)
        n83 = Greater?(x=w227, y="10 Min") -> (0:w225:bool)
        "15 min Up" <- w225
        n84 = case shown="True" w225 {
          selector: w225 -> [w236 _]
          tunnel: [w236 w237] -> w224
          tunnel: w223 -> [_ w244]
          frame False {
          }
          frame True {
            n85 = Delete From Array(array=w244, length=600) -> (deleted portion=w242:dbl[])  [unwired: 1 in, 1 out]
            n86 = Array Max & Min(array=w242) -> (max value=w241:dbl, min value=w240:dbl)  [unwired: 2 out]
            n87 = Subtract(x=w241, y=w240) -> (x-y=w239:dbl)
            n88 = Less?(x=w239, y=2.0) -> (x < y?=w237:bool)
          }
        }
        "Temp stable" <- w224
        n89 = case shown="False" w224 {
          tunnel: w232 -> [w253 w260]
          tunnel: [w252 w260] -> w231
          tunnel: [w250 "" ("State(s) in Front (\"\")")] -> w230
          tunnel: w229 -> [_ _]
          tunnel: w223 -> [w247 _]
          frame False {
            n90 = call "UTILITY E-Time.vi"() -> ("Elapsed Time (sec)"=w245:dbl)  [unwired: 9 in, 2 out]
            n91 = call "UTILITY Timeout Calc.vi"("Timer"=w245, "Gather Data Period"=1000) -> ("coerced(x)"=w249:i32)  [unwired: 8 in, 1 out]
            n92 = event shown="[0] Timeout" {
              selector: _ -> [_]
              dyn-events: _ -> [_]
              timeout: w249 -> [_]
              tunnel: [w258] -> w251
              tunnel: ["Post Time\nGet Power\nCDAQ: Get Data\nWait for Temp Stable for 10 Min" ("State(s) in Front (\"\")")] -> w250
              tunnel: w247 -> [w256]
              tunnel: [w255] -> w246
              event Timeout {
                n93 = event-data() -> ()  [unwired: 1 in, 2 out]
                n94 = local read "RDB F"() -> (w254:dbl)
                n95 = call "UTILITY E-Time.vi"() -> ("Elapsed Time (sec)"=w258:dbl)  [unwired: 9 in, 2 out]
                n96 = Build Array (concatenate)(w256, w254) -> (w255:dbl[])
              }
            }
            "Tstart 10min" <- w251
            n97 = Bundle By Name(cluster=w253, "Tstart"=w251, "Temps"=w246) -> (w252:T13)
          }
          frame True {
          }
        }
        n98 = local write "Board ID"("Air Fluffing...") -> ()
        n99 = call <vilib>:"Add State(s) to Queue__jki_lib_state_machine.vi"("State(s) in Front (\"\")"=w230, "State(s) in (\"\")"=w235) -> ("States Out"=w234:string)  [unwired: 13 in]
      }
      frame "-----------Equipment--------------" {
        n100 = call <vilib>:"Add State(s) to Queue__jki_lib_state_machine.vi"("State(s) in (\"\")"=w264) -> ("States Out"=w263:string)  [unwired: 14 in]
      }
      frame "Init: Time" {
        n101 = call "UTILITY E-Time.vi"("error in (no error)"=w265) -> ("error out"=w267:errorcluster, "Elapsed Time (sec)"=w268:dbl)  [unwired: 8 in, 1 out]
        n102 = Bundle By Name(cluster=w266, "T0"=w268, "Tstart"=w268) -> (w269:T13)
        n103 = call <vilib>:"Add State(s) to Queue__jki_lib_state_machine.vi"("State(s) in (\"\")"=w271) -> ("States Out"=w270:string)  [unwired: 14 in]
      }
      frame "Get Power" {
        # "WT500 Visa"
        n104 = Unbundle By Name(w277) -> ("Test Fixture Hardware.Power.Yokogawa.WT500.Power VISA Yokogawa WT500"=w274:refnum<visa-resource-name>)
        n105 = call "WT500 Get Power Data.vi"("Error In"=w273, "VISA resource name"=w274) -> ("Error Out"=w272:errorcluster, "Power Data Out"=w275:T15)  [unwired: 3 in, 4 out]
        n106 = Unbundle By Name(w275) -> ("Power (W):Sigma"=→"Power (Watts)":dbl)
        n107 = call <vilib>:"Add State(s) to Queue__jki_lib_state_machine.vi"("State(s) in (\"\")"=w279) -> ("States Out"=w278:string)  [unwired: 14 in]
      }
      frame "CDAQ: Get Data" {
        n108 = Unbundle By Name(w297) -> ("Test Fixture Hardware.Analog Data.NI Tasks (Dryer DOE)"=w296:refnum<k21>[], "Test Fixture Hardware.ITHX-Temp Humidity.IP Address 1"=w284:string, "Test Fixture Hardware.ITHX-Temp Humidity.Remote Port"=w283:u16)
        n109 = call "DPT GET NI Data.vi"("NI Card Settings"=T12 {"Disable NI Card 1"=FALSE, "Disable NI Card 2"=TRUE, "Disable NI Card 3"=TRUE, "Disable NI Card 4"=TRUE, "Disable NI Card 5"=TRUE, "Disable NI Card 6"=TRUE, "Disable NI Card 7"=FALSE}, "Error In"=w295, "Tasks In"=w296) -> ("Error Out"=w289:errorcluster, "cDAQ Data"=w294:string[][])  [unwired: 7 in]
        n110 = Index Array(array=w294, index (row)=0 ("disabled index (row)"), index (col)=1 ("disabled index (col)")) -> (element=w291:string)
        n111 = call "Newport ITX-D3N.vi"("Disable Filter?"=TRUE, "Device Number (Display In Header)"="1", "error in (no error)"=w289, "Remote Port"=w283, "Machine"=w284) -> ("error out"=w288:errorcluster, "iTHX/iBTHX Output"=w287:T16)  [unwired: 3 in, 2 out]
        n112 = Fract/Exp String To Number(string=w291) -> (number=→"TC 1 - RDB (°F)" →"RDB F":dbl)  [unwired: 3 in, 1 out]
        n113 = Unbundle By Name(w287) -> ("iBTHX Temperature (°F)"=→"Ambient Temp(F)":dbl, "iBTHX Humidity (%)"=→"Relative Humidity":dbl)
        n114 = call <vilib>:"Add State(s) to Queue__jki_lib_state_machine.vi"("State(s) in (\"\")"=w299) -> ("States Out"=w298:string)  [unwired: 14 in]
      }
      frame "Post Time" {
        n115 = Unbundle By Name(w304) -> ("T0"=w302:dbl)
        "T0" <- w302
        n116 = call "UTILITY E-Time.vi"() -> ("Elapsed Time (sec)"=w303:dbl)  [unwired: 9 in, 2 out]
        n117 = Subtract(x=w303, y=w302) -> (x-y=→"Timer":dbl)
        n118 = call <vilib>:"Add State(s) to Queue__jki_lib_state_machine.vi"("State(s) in (\"\")"=w306) -> ("States Out"=w305:string)  [unwired: 14 in]
      }
      frame "Get Cold Dryer Weight" {
        n119 = Unbundle By Name(w307) -> ("Test Fixture Hardware.Weight Scale.Select Scale"=w311:string)
        n120 = case shown="\"IND560 SERIAL\"" w311 {
          tunnel: w307 -> [w317 w327]
          tunnel: [w319 w325] -> w310
          tunnel: w309 -> [w321 w324]
          tunnel: [w320 w323] -> w313
          tunnel: FALSE ("Use While Loop?") -> [w318 w322]
          frame "IND560 SERIAL" {
            n121 = Unbundle By Name(w317) -> ("Test Fixture Hardware.Weight Scale.Com Options.IND560Scale VISA"=w316:refnum<visa-resource-name>)
            n122 = call "IND560 Serial Tester.vi"("Use While Loop?"=w318, "Error In"=w321, "VISA Input"=w316) -> ("Error Out"=w320:errorcluster, "Net Weight"=w319:dbl)  [unwired: 7 in]
          }
          frame "GSE 350", Default {
            n123 = Unbundle By Name(w327) -> ("Test Fixture Hardware.Weight Scale.Com Options.GSE 350"=w326:refnum<visa-resource-name>)
            n124 = call "GSE 350 Main.vi"("Use While Loop?"=w322, "Error In"=w324, "VISA Refnum in"=w326) -> ("Error Out"=w323:errorcluster, "Weight (lb/kg)"=w325:dbl)  [unwired: 6 in, 1 out]
          }
        }
        "Cold Dryer Weight" <- w310
        n125 = call <vilib>:"Clear Errors.vi"("error in (no error)"=w313) -> ("error out"=w308:errorcluster)  [unwired: 5 in, 1 out]
        n126 = call <vilib>:"Add State(s) to Queue__jki_lib_state_machine.vi"("State(s) in (\"\")"=w315) -> ("States Out"=w314:string)  [unwired: 14 in]
      }
    }
    n127 = case shown="True" "Debug?" {
      tunnel: w11 -> [_ w25]
      tunnel: w9 -> [w22 w24]
      tunnel: [w22 w23] -> w10
      frame False {
      }
      frame True {
        n128 = Build Array (concatenate)(w24, w25) -> (w23:string[])
        "Debug State" <- w23
      }
    }
  }
  "Error Out" <- w2
